vi "onMouseDown.vi"(8 "error in (no error)":errorcluster, 10 "Invert":bool, 11 "Filled Text Fields Actor in":refnum<class "Filled Text Fields Actor.lvclass">) -> (0 "error out":errorcluster, 3 "Filled Text Fields Actor out":refnum<class "Filled Text Fields Actor.lvclass">)   [LabVIEW 2017, in "Filled Text Fields.lvlib" / "Filled Text Fields Actor.lvclass"]
uses:
  Filled Text Fields Actor.lvclass
  Filled Text Fields Actor.lvclass/Filled Text Fields Actor.ctl
  Filled Text Fields.States.ctl
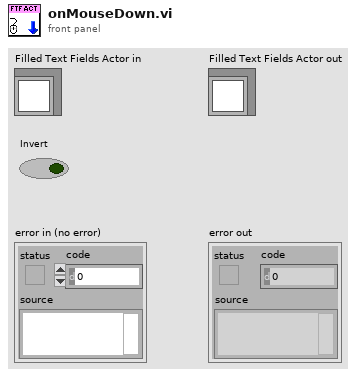
[diagram p1: front panel]
types:
  T1 = typedef "Filled Text Fields.lvlib/Filled Text Fields Actor.lvclass/Filled Text Fields.States.ctl" = enum16{"Inactive", "Activated", "Error", "Focused", "Hover", "Disabled", "Disabled and Grey out"}
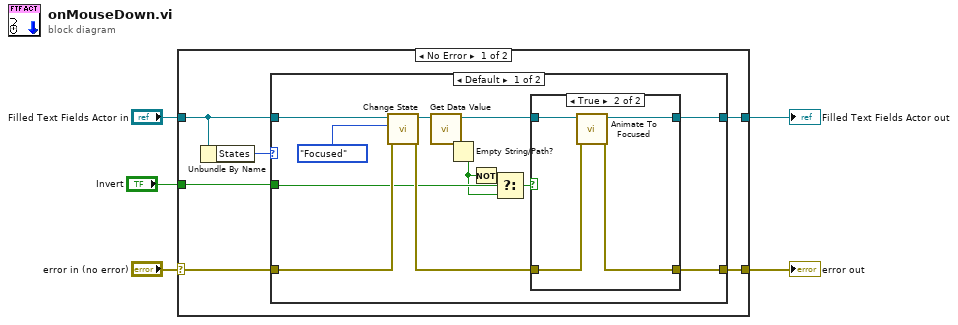
[diagram p0: block diagram]
diagram:
  n1 = case shown="No Error" "error in (no error)" {
    selector: "error in (no error)" -> [w10 w34]
    tunnel: [w9 w34] -> w3
    tunnel: [w11 w33] -> w4
    tunnel: "Filled Text Fields Actor in" -> [w8 w33]
    tunnel: "Invert" -> [w6 _]
    frame No Error {
      n2 = Unbundle By Name(w8) -> ("States"=w7:T1)
      n3 = case shown="Default" w7 {
        tunnel: [w18 w32] -> w11
        tunnel: w10 -> [w23 w31]
        tunnel: [w16 w31] -> w9
        tunnel: w8 -> [w21 w32]
        tunnel: w6 -> [w15 _]
        frame Default {
          n4 = call "Change State.vi"("error in (no error)"=w23, "New State"=Filled_Text_Fields.States."Focused", "Filled Text Fields Actor in"=w21) -> ("error out"=w17:errorcluster, "Filled Text Fields Actor out"=w24:refnum<class "Filled Text Fields Actor.lvclass">)  [unwired: 7 in]
          n5 = call "Get Data Value.vi"("Filled Text Fields Actor in"=w24) -> ("Value"=w20:string, "Filled Text Fields Actor out"=w19:refnum<class "Filled Text Fields Actor.lvclass">)  [unwired: 9 in]
          n6 = Empty String/Path?(string/path=w20) -> (empty?=w14:bool)
          n7 = Not(x=w14) -> (.not. x?=w12:bool)
          n8 = Select(t=w12, s=w15, f=w14) -> (s? t:f=w13:bool)
          n9 = case shown="True" w13 {
            tunnel: w19 -> [w26 w30]
            tunnel: [w26 w29] -> w18
            tunnel: w17 -> [w25 w28]
            tunnel: [w25 w27] -> w16
            frame False {
            }
            frame True {
              n10 = call "Animate To Focused.vi"("error in (no error)"=w28, "Filled Text Fields Actor in"=w30) -> ("error out"=w27:errorcluster, "Filled Text Fields Actor out"=w29:refnum<class "Filled Text Fields Actor.lvclass">)  [unwired: 8 in]
            }
          }
        }
        frame "Focused" {
        }
      }
    }
    frame Error {
    }
  }
  "error out" <- w3
  "Filled Text Fields Actor out" <- w4
